vi "FetchAllDbl.vi"(8 "error in (no error)":errorcluster, 11 "DigitizerBase in":refnum<class "DigitizerBase.lvclass">) -> (0 "error out":errorcluster, 3 "DigitizerBase out":refnum<class "DigitizerBase.lvclass">)   [LabVIEW 2014, in "DigitizerPlugins.lvlib" / "DigitizerBase.lvclass"]
uses:
  DigitizerBase.lvclass
  DigitizerBase.lvclass/DigitizerBase.ctl
  Typedefs/WfrmAttributes.ctl
  Accessors/Read Waveforms.vi
  Accessors/Write Waveforms.vi
  Accessors/Read InstRef.vi
  Accessors/Read Channels.vi
  Accessors/Read Acquisition.vi
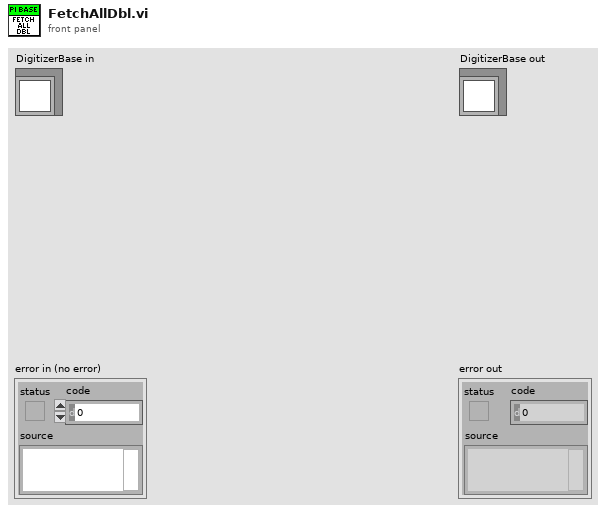
[diagram p1: front panel]
types:
  T1 = typedef "DigitizerPlugins.lvlib/DigitizerBase.lvclass/WfrmAttributes.ctl" = cluster{"XOffset":dbl, "ActualPts":i64, "FirstValid":i64}
  T2 = typedef "DigitizerPlugins.lvlib/DigitizerBase.lvclass/Channel.ctl" = cluster{"Name":string, "Enabled":bool, "InputImpedance":dbl, "Coupling":enum16{"AC", "DC", "Gnd"}, "Offset":dbl, "Range":dbl}
  T3 = typedef "DigitizerPlugins.lvlib/DigitizerBase.lvclass/Acquisition.ctl" = cluster{"SampleRate":dbl, "RecordSize":i32, "NumRecords":i32, "SampleMode":i32, "Timeout (ms)":i32}
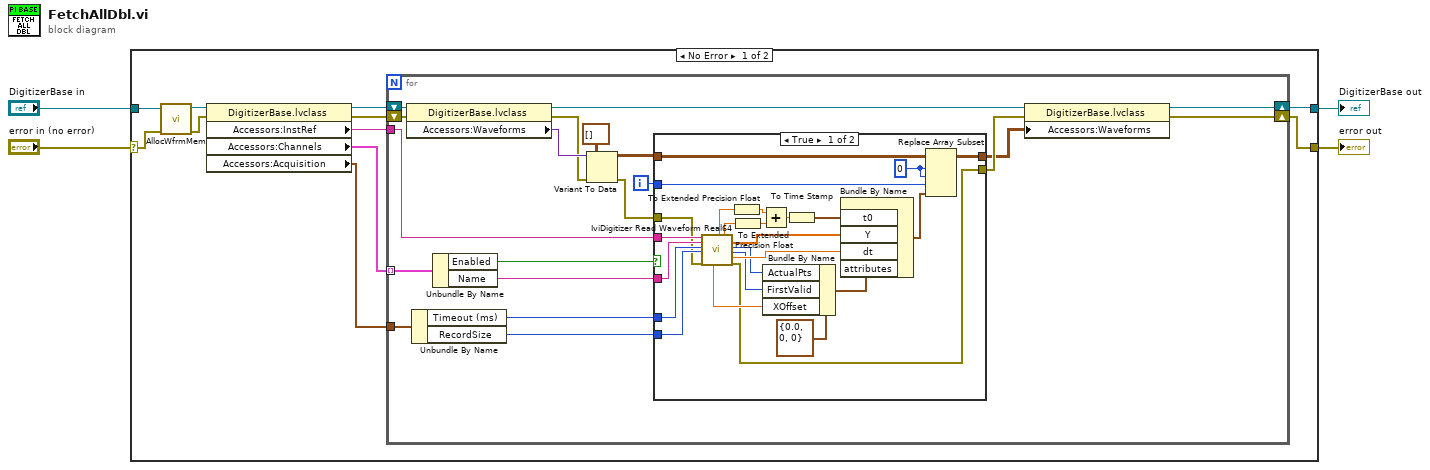
[diagram p0: block diagram]
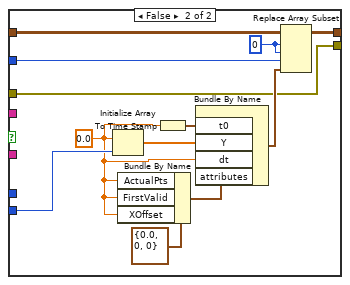
[diagram p2: hidden frame]
diagram:
  n1 = case shown="No Error" "error in (no error)" {
    selector: "error in (no error)" -> [w14 w73]
    tunnel: [w5 w73] -> w3
    tunnel: [w6 w72] -> w1
    tunnel: "DigitizerBase in" -> [w15 w72]
    frame No Error {
      n2 = call-dynamic "AllocWfrmMem.vi"("error in (no error)"=w14, "DigitizerBase in"=w15) -> ("error out"=w7:errorcluster, "DigitizerBase out"=w13:refnum<class "DigitizerBase.lvclass">)  [unwired: 8 in]
      n3 = property class="DigitizerBase.lvclass"(reference=w13, error in=w7) -> (reference out=w11:refnum<class "DigitizerBase.lvclass">, error out=w10:errorcluster, "Accessors:InstRef"=w12:string, "Accessors:Channels"=w9:T2[], "Accessors:Acquisition"=w8:T3)
      n4 = for {
        tunnel: w12 -> [w29]
        tunnel: w9 -> [w35] mode=indexing
        tunnel: w8 -> [w31]
        shift-right: [w17] -> w6
        shift-left: w11 -> [w33]
        shift-right: [w16] -> w5
        shift-left: w10 -> [w34]
        i -> [w26]
        n5 = property class="DigitizerBase.lvclass"(reference=w33, error in=w34) -> (reference out=w20:refnum<class "DigitizerBase.lvclass">, error out=w22:errorcluster, "Accessors:Waveforms"=w24:variant)
        n6 = Unbundle By Name(w31) -> ("Timeout (ms)"=w28:i32, "RecordSize"=w27:i32)
        n7 = Unbundle By Name(w35) -> ("Enabled"=w32:bool, "Name"=w30:string)
        n8 = Variant To Data(error in=w22, type=waveform(dbl)[][][] [], Variant=w24) -> (data=w23:waveform(dbl)[][][], error out=w21:errorcluster)
        n9 = case shown="True" w32 {
          tunnel: w30 -> [w58 _]
          tunnel: w29 -> [w59 _]
          tunnel: w28 -> [w57 _]
          tunnel: w27 -> [w56 w64]
          tunnel: w26 -> [w55 w71]
          tunnel: [w39 w66] -> w18
          tunnel: [w38 w60] -> w19
          tunnel: w23 -> [w37 w65]
          tunnel: w21 -> [w36 w60]
          frame True {
            w45 = 0 ("index (page)")
            n10 = call <vilib>:"IviDigitizer Read Waveform Real64.vi"("instrument handle"=w59, "Channel Name (\"\")"=w58, "Maximum Time (5000)"=w57, "Waveform Array Size (256)"=w56, "error in (no error)"=w36) -> ("Initial X Offset"=w43:dbl, "Initial X Time Seconds"=w48:dbl, "Initial X Time Fraction"=w54:dbl, "Waveform Array"=w49:dbl[], "Actual Points"=w42:i64, "First Valid Point"=w41:i64, "X Increment"=w47:dbl, "error out"=w38:errorcluster)  [unwired: 6 in, 1 out]
            n11 = To Extended Precision Float(1:w48) -> (0:w53:ext)
            n12 = To Extended Precision Float(1:w54) -> (0:w52:ext)
            n13 = Add(x=w53, y=w52) -> (x+y=w51:ext)
            n14 = Bundle By Name(cluster=T1 {"XOffset"=0.0, "ActualPts"=0, "FirstValid"=0} ("Attributes"), "ActualPts"=w42, "FirstValid"=w41, "XOffset"=w43) -> (w40:T1)
            n15 = To Time Stamp(1:w51) -> (0:w50:timestamp)
            n16 = Bundle By Name("t0"=w50, "Y"=w49, "dt"=w47, "attributes"=w40) -> (w46:waveform(dbl))  [unwired: 1 in]
            n17 = Replace Array Subset(array=w37, new element=w46, index (dim 0)=w45, index (dim 1)=w45, index (dim 2)=w55) -> (w39:waveform(dbl)[][][])
          }
          frame False {
            w61 = 0.0 ("element")
            w69 = 0 ("index (page)")
            n18 = Initialize Array(w61, w64) -> (w63:dbl[])
            n19 = Bundle By Name(cluster=T1 {"XOffset"=0.0, "ActualPts"=0, "FirstValid"=0} ("Attributes"), "ActualPts"=w61, "FirstValid"=w61, "XOffset"=w61) -> (w67:T1)
            n20 = To Time Stamp(1:w61) -> (0:w62:timestamp)
            n21 = Bundle By Name("t0"=w62, "Y"=w63, "dt"=w61, "attributes"=w67) -> (w70:waveform(dbl))  [unwired: 1 in]
            n22 = Replace Array Subset(array=w65, new element=w70, index (dim 0)=w69, index (dim 1)=w69, index (dim 2)=w71) -> (w66:waveform(dbl)[][][])
          }
        }
        n23 = property class="DigitizerBase.lvclass"(reference=w20, error in=w19, "Accessors:Waveforms"=w18) -> (reference out=w17:refnum<class "DigitizerBase.lvclass">, error out=w16:errorcluster)
      }
    }
    frame Error {
    }
  }
  "error out" <- w3
  "DigitizerBase out" <- w1
